vi "Trab_V1.vi"() -> ()   [LabVIEW 2020]
uses:
  <vilib>/measure/NI_MABase.lvlib
panel:
  in  "?":T1={"Taxa de Amostragem"=1000.0, "Número de Amostras"=10000.0} {"Número de Amostras" format="%#.6g"; "Taxa de Amostragem" format="%#.6g"}
  out "Erro:":string
  in  "C - Capacitância":dbl
  in  "L -  Indutância":dbl
  in  "Boolean":bool
  in  "?":i32(knob) scale=0.0..2.0
  out "Onda de Entrada:":waveform(dbl)(graph)
  in  "R - Resistência":dbl
  in  "Amplitude":dbl
  in  "Duty Cicle":dbl
  in  "Frequência":dbl
  # "SIMULADOR RLC"
  # "Onda Senoidal"
  # "Onda Quadrada"
  # "Onda de um Arquivo"
  # "Verde=Continuar While"
  # "Preto=Pausar While"
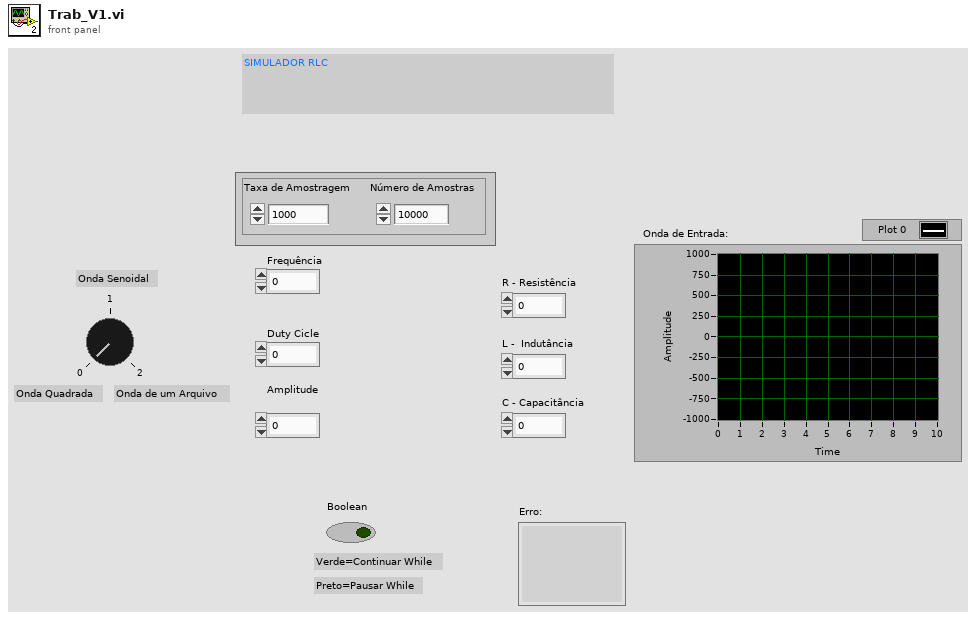
[diagram p1: front panel]
types:
  T1 = cluster{"Taxa de Amostragem":dbl, "Número de Amostras":dbl}
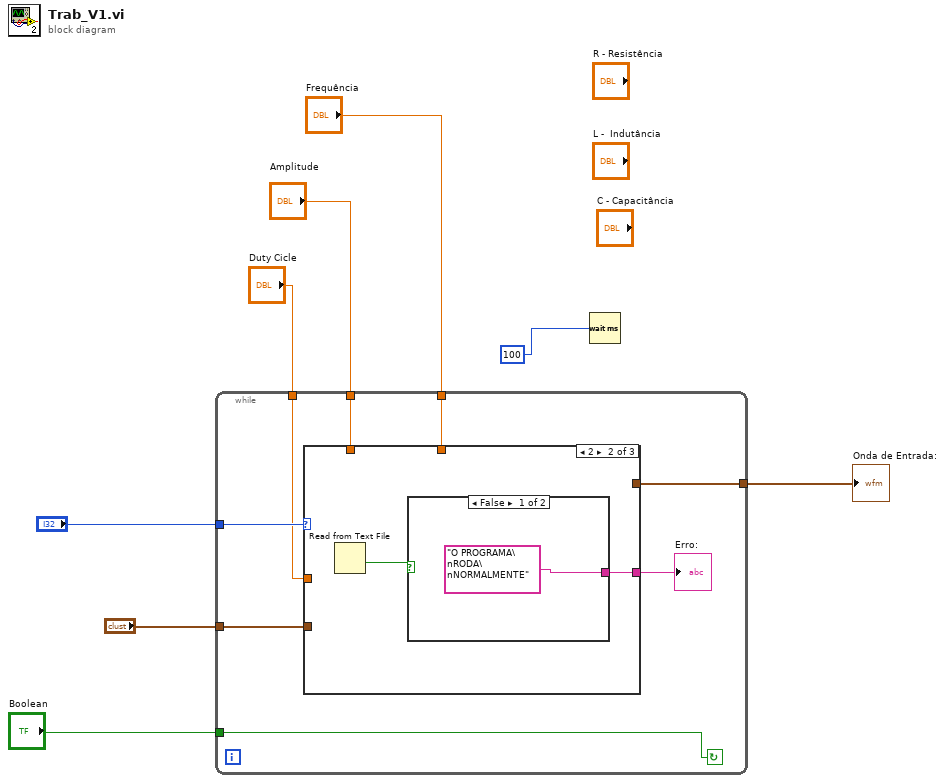
[diagram p0: block diagram]
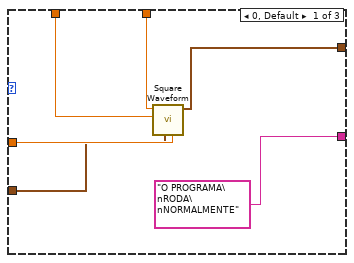
[diagram p2: hidden frame]
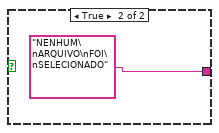
[diagram p3: hidden frame]
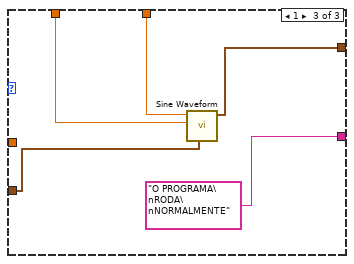
[diagram p4: hidden frame]
diagram:
  n1 = while {
    tunnel: "?" -> [w16]
    tunnel: "Boolean" -> [w15]
    tunnel: "Amplitude" -> [w14]
    tunnel: "Frequência" -> [w13]
    tunnel: "Duty Cicle" -> [w12]
    tunnel: [w10] -> w2
    tunnel: "?" -> [w9]
    stop <- w15 continue-if-true
    n2 = case shown="2" w16 {
      tunnel: w14 -> [w22 _ w30]
      tunnel: w13 -> [w21 _ w31]
      tunnel: w12 -> [w20 _ _]
      tunnel: ["O PROGRAMA\nRODA\nNORMALMENTE" w23 "O PROGRAMA\nRODA\nNORMALMENTE"] -> w11
      tunnel: [w18 _ w28] -> w10
      tunnel: w9 -> [w17 _ w27]
      frame 0, Default {
        n3 = call <vilib>:"Square Waveform.vi"("duty cycle (%)"=w20, "sampling info"=w17, "amplitude"=w22, "frequency"=w21) -> ("signal out"=w18:waveform(dbl))  [unwired: 6 in, 1 out]
      }
      frame 2 {
        n4 = Read from Text File() -> (cancelled=w24:bool)  [unwired: 4 in, 3 out]
        n5 = case shown="False" w24 {
          tunnel: ["O PROGRAMA\nRODA\nNORMALMENTE" "NENHUM\nARQUIVO\nFOI\nSELECIONADO"] -> w23
          frame False {
          }
          frame True {
          }
        }
      }
      frame 1 {
        n6 = call <vilib>:"Sine Waveform.vi"("sampling info"=w27, "amplitude"=w30, "frequency"=w31) -> ("signal out"=w28:waveform(dbl))  [unwired: 7 in, 1 out]
      }
    }
    "Erro:" <- w11
  }
  "Onda de Entrada:" <- w2
  n7 = Wait (ms)(milliseconds to wait=u32 100) -> ()  [unwired: 1 out]
